vi "Prepare Firmware.vi"(2 "error in":errorcluster, 3 "Firmware file":path) -> (0 "error out":errorcluster, 1 "data":u8[][](array[numeric]))   [LabVIEW 2010]
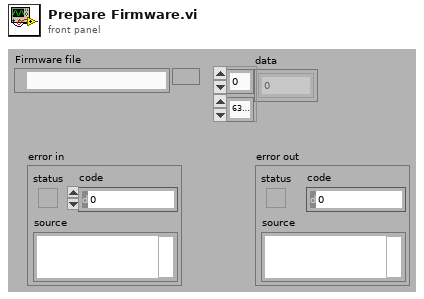
[diagram p1: front panel]
types:
  T1 = enum16{"big-endian, network order", "native, host order", "little-endian"}
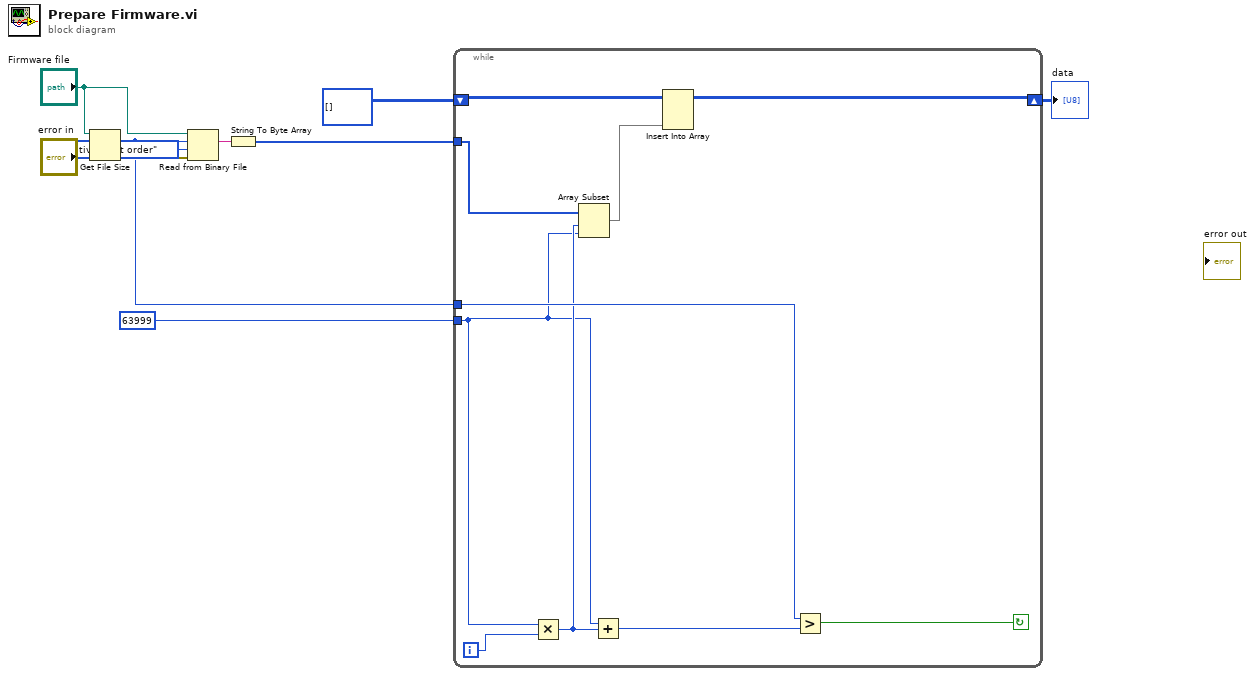
[diagram p0: block diagram]
diagram:
  n1 = Get File Size(file="Firmware file", error in="error in") -> (size (in bytes)=w6:i64, 0:w8:errorcluster)  [unwired: 1 out]
  n2 = Read from Binary File(8:w8, 9:T1."native, host order" ("byte order (0:big-endian, network order)"), 10:w6, 11:"Firmware file") -> (2:w5:string)  [unwired: 2 in, 3 out]
  n3 = String To Byte Array(string=w5) -> (unsigned byte array=w4:u8[])
  n4 = while {
    tunnel: 63999 ("Numeric") -> [w14]
    tunnel: w6 -> [w19]
    tunnel: w4 -> [w17]
    shift-right: [w11] -> w2
    shift-left: u8[][] [] ("unsigned byte array") -> [w13]
    i -> [w20]
    stop <- w18 continue-if-true
    n5 = Multiply(x=w14, y=w20) -> (x*y=w16:i32)
    n6 = Array Subset(array=w17, index=w16, length=w14) -> (w12:u8[])
    n7 = Add(x=w14, y=w16) -> (x+y=w15:i32)
    n8 = Insert Into Array(array=w13, new element=w12) -> (w11:u8[][])  [unwired: 2 in]
    n9 = Greater?(x=w19, y=w15) -> (0:w18:bool)
  }
  "data" <- w2
